vi "GetTDs&SpecRs.vi"(8 "error in":errorcluster) -> (0 "error out":errorcluster, 3 "TDSegArray":string[][](array[string]))   [LabVIEW 2012]
uses:
  bin/OVA32.dll
panel:
  out "segTD":string
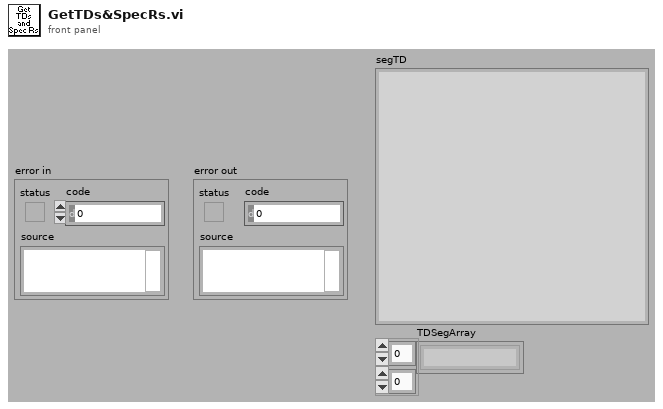
[diagram p1: front panel]
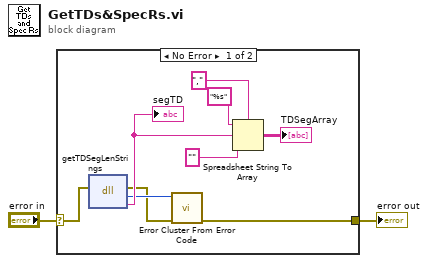
[diagram p0: block diagram]
diagram:
  n1 = case shown="No Error" "error in" {
    selector: "error in" -> [w7 w12]
    tunnel: [w3 w12] -> w2
    frame No Error {
      n2 = dll-call lib="C:/_src/OVA5000_DSP_falcon/Software/LabVIEW/OVA/SDK/OVA_5000_SDK_v5.14.3/bin/OVA32.dll" fn="getTDSegLenStrings"(error in=w7) -> (error out=w4:errorcluster, "return type"=w5:i32, "segTD"=w6:string)  [unwired: 3 in, 1 out]
      "segTD" <- w6
      n3 = call <vilib>:"Error Cluster From Error Code.vi"("error in (no error)"=w4, "error code (0)"=w5) -> ("error out"=w3:errorcluster)  [unwired: 7 in]
      n4 = Spreadsheet String To Array(delimiter (Tab)=",", format string="%s", spreadsheet string=w6, array type (2D Dbl)="") -> (array=→"TDSegArray":string[][])
    }
    frame Error {
    }
  }
  "error out" <- w2
